vi "Permanentbereich aufrufen.vi"(10 "Permanent (Eingang)":refnum<vi>, 11 "VI (Eingang)":refnum<vi>) -> (2 "Permanent (Ausgang)":refnum<vi>, 3 "VI (Ausgang)":refnum<vi>)   [LabVIEW 2020, in "Bildwechsel.lvlib"]
uses:
  Bildwechsel.lvlib
  Allgemein/allgemeine Sub-VIs.lvlib
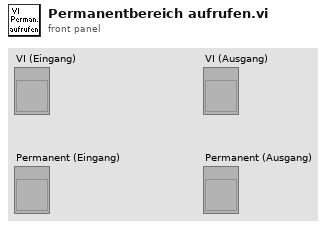
[diagram p1: front panel]
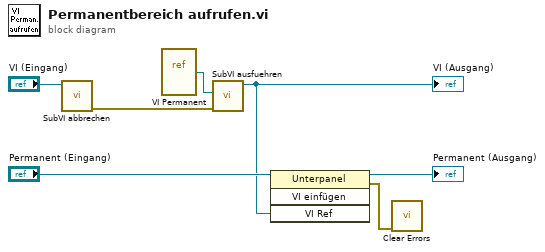
[diagram p0: block diagram]
diagram:
  n1 = call "SubVI abbrechen.vi"("vi reference"="VI (Eingang)") -> ("error out"=w1:errorcluster)  [unwired: 1 in, 5 out]
  n2 = vi-ref "VI Permanent.vi"() -> (w3:refnum<vi>)
  n3 = call "SubVI ausfuehren.vi"("Fehler"=w1, "Referenz"=w3) -> ("vi reference"=w5:refnum<vi>)  [unwired: 9 in]
  "VI (Ausgang)" <- w5
  n4 = invoke on="Methodenknoten" class="Unterpanel" method="VI einfügen"(reference="Permanent (Eingang)", "VI Ref"=w5) -> (reference out=→"Permanent (Ausgang)":refnum<vi>, error out=w2:errorcluster)  [unwired: 2 in, 2 out]
  n5 = call <vilib>:"Clear Errors.vi"("error in (no error)"=w2) -> ()  [unwired: 5 in, 2 out]
